vi "Piezo wiggle.vi"() -> ()   [LabVIEW 2017]
panel:
  in  "Amplitude":dbl=37.5 min=0.0 max=75.0
  in  "Frequency (Hz)":dbl=1.0
  out "error out":errorcluster
  in  "stop":bool
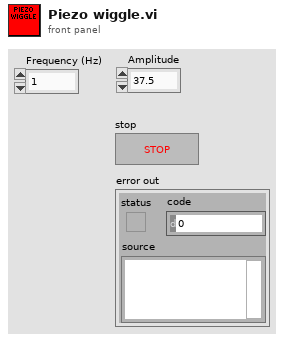
[diagram p1: front panel]
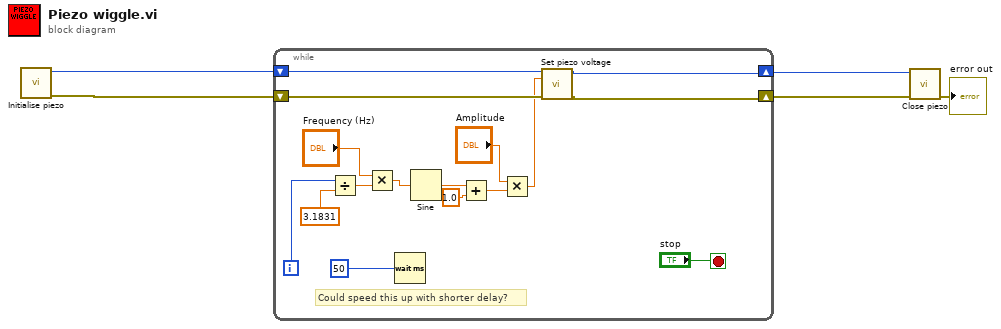
[diagram p0: block diagram]
diagram:
  n1 = call "Initialise piezo.vi"() -> ("Piezo error out"=w2:errorcluster, "Piezo handle"=w1:i32)  [unwired: 10 in]
  n2 = while {
    shift-right: [w13] -> w5
    shift-left: w1 -> [w12]
    shift-right: [w14] -> w4
    shift-left: w2 -> [w11]
    i -> [w19]
    stop <- "stop" stop-if-true
    # "Could speed this up with shorter delay?"
    n3 = Divide(x=w19, y=3.1831) -> (x/y=w10:dbl)
    n4 = Multiply(x="Frequency (Hz)", y=w10) -> (x*y=w9:dbl)
    n5 = Wait (ms)(milliseconds to wait=u32 50) -> ()  [unwired: 1 out]
    n6 = Sine(x=w9) -> (sin(x)=w17:dbl)
    n7 = Add(x=w17, y=1.0) -> (x+y=w15:dbl)
    n8 = Multiply(x="Amplitude", y=w15) -> (x*y=w7:dbl)
    n9 = call "Set piezo voltage.vi"("Piezo handle"=w12, "X Voltage"=w7, "Piezo error in"=w11) -> ("Piezo handle out"=w13:i32, "Piezo error out"=w14:errorcluster)  [unwired: 11 in]
  }
  n10 = call "Close piezo.vi"("Piezo error in"=w4, "Piezo handle"=w5) -> ("error out"=→"error out":errorcluster)  [unwired: 9 in]
